vi "Write Name Specs.vi"(10 "Name Specs":refnum<class "Name Specs.lvclass">, 11 "Rescript in":refnum<class "_Rescript.lvclass">) -> (3 "_Rescript out":refnum<class "_Rescript.lvclass">)   [LabVIEW 2020, in "_Rescript.lvlib" / "_Rescript.lvclass"]
uses:
  _Rescript.lvclass
  _Shared/Name Specs/Name Specs.lvclass
  _Rescript.lvclass/_Rescript.ctl
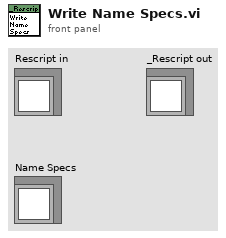
[diagram p1: front panel]
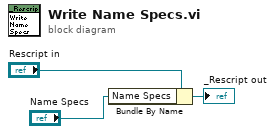
[diagram p0: block diagram]
diagram:
  n1 = Bundle By Name(cluster="Rescript in", "Name Specs"="Name Specs") -> (→"_Rescript out":refnum<class "_Rescript.lvclass">)
